vi "HostSpeedCalc (1).vi"(9 "Period (ms)":u32, 10 "Distance (m)":dbl) -> (2 "Speed (cm/s)":u32)   [LabVIEW 2017]
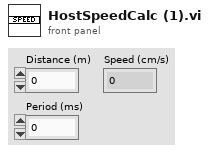
[diagram p1: front panel]
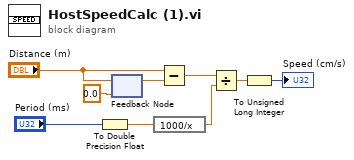
[diagram p0: block diagram]
diagram:
  n1 = To Double Precision Float(number="Period (ms)") -> (double precision float=w2:dbl)
  n2 = feedback-in #1("Distance (m)") -> ()
  n3 = feedback #1(0.0 ("Distance (m)")) -> (w9:dbl)
  n4 = expression code="1000/x"(w2) -> (w1:dbl)
  n5 = Subtract(x="Distance (m)", y=w9) -> (x-y=w7:dbl)
  n6 = Divide(x=w7, y=w1) -> (x/y=w4:dbl)
  n7 = To Unsigned Long Integer(number=w4) -> (unsigned 32bit integer=→"Speed (cm/s)":u32)
